vi "LidarROI.vi"(0 "x,y 배열":cluster{"x":dbl, "y":dbl}[](array[cluster])) -> (4 "ROI1":bool, 6 "ROI2":bool, 8 "ROI3":bool, 10 "왼쪽정적라이다스티어":dbl=144.0774265029782, 15 "오른쪽정적라이다스티어":dbl=-108.05806987723365)   [LabVIEW 2015]
panel:
  in  "x 场2":dbl=-100.0
  in  "y시작 3":dbl=500.0
  in  "y场 3":dbl=3000.0
  in  "x场 3":dbl=1400.0
  in  "x시작 3":dbl=100.0
  in  "x시작 2":dbl=-1400.0
  in  "y场 2":dbl=3000.0
  in  "y시작 2":dbl=500.0
  in  "x시작":dbl=-1400.0
  in  "x场":dbl=1400.0
  in  "y场":dbl=8000.0
  in  "y시작":dbl
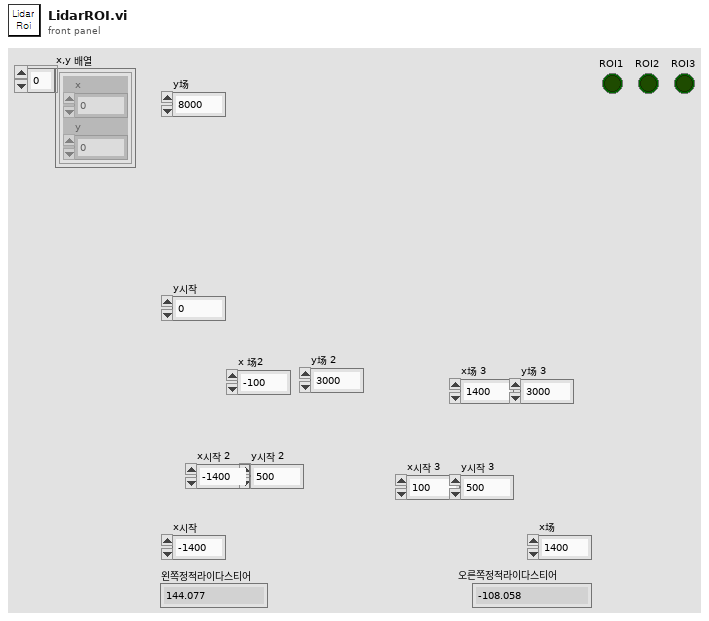
[diagram p1: front panel]
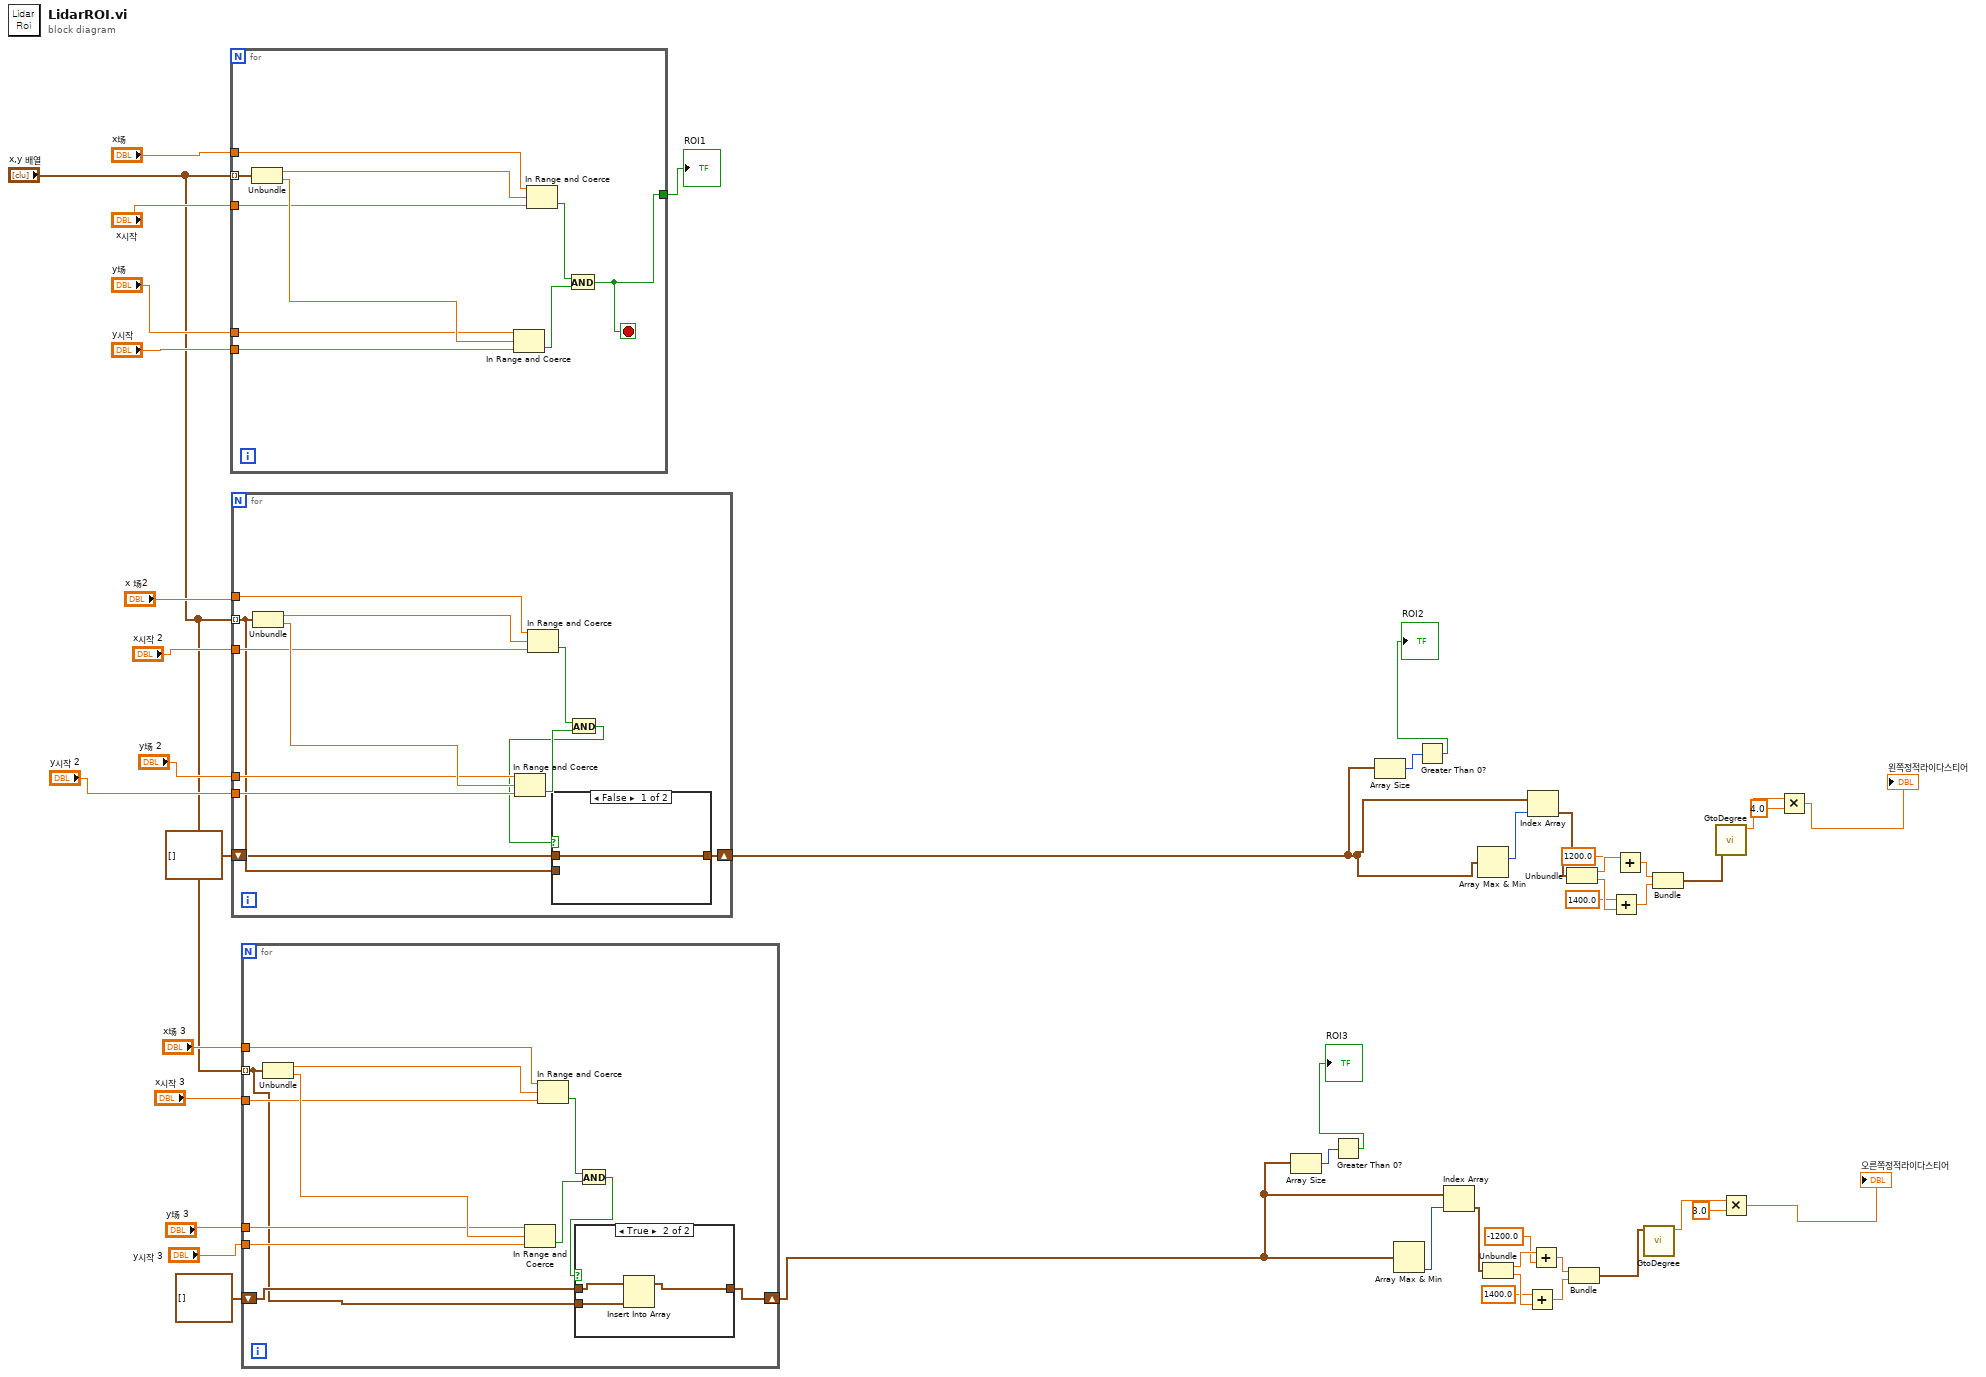
[diagram p0: block diagram]
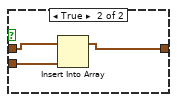
[diagram p3: hidden frame]
diagram:
  n1 = for {
    tunnel: "x,y 배열" -> [w56] mode=indexing
    tunnel: [w51] -> w46
    tunnel: "x场" -> [w50]
    tunnel: "x시작" -> [w49]
    tunnel: "y场" -> [w48]
    tunnel: "y시작" -> [w47]
    stop <- w51 stop-if-true
    n2 = Unbundle(w56) -> ("x"=w55:dbl, "y"=w52:dbl)
    n3 = In Range and Coerce(upper limit=w48, x=w52, lower limit=w47) -> (In Range?=w53:bool)  [unwired: 1 out]
    n4 = In Range and Coerce(upper limit=w50, x=w55, lower limit=w49) -> (In Range?=w54:bool)  [unwired: 1 out]
    n5 = And(x=w54, y=w53) -> (x .and. y?=w51:bool)
  }
  "ROI1" <- w46
  n6 = for {
    tunnel: "x,y 배열" -> [w59] mode=indexing
    tunnel: "x 场2" -> [w64]
    tunnel: "x시작 2" -> [w63]
    tunnel: "y场 2" -> [w62]
    tunnel: "y시작 2" -> [w61]
    shift-right: [w58] -> w31
    shift-left: cluster{"x":dbl, "y":dbl}[] [] -> [w57]
    n7 = Unbundle(w59) -> ("x"=w68:dbl, "y"=w65:dbl)
    n8 = In Range and Coerce(upper limit=w62, x=w65, lower limit=w61) -> (In Range?=w66:bool)  [unwired: 1 out]
    n9 = In Range and Coerce(upper limit=w64, x=w68, lower limit=w63) -> (In Range?=w67:bool)  [unwired: 1 out]
    n10 = And(x=w67, y=w66) -> (x .and. y?=w60:bool)
    n11 = case shown="False" w60 {
      tunnel: w59 -> [_ w72]
      tunnel: [w69 w71] -> w58
      tunnel: w57 -> [w69 w70]
      frame False {
      }
      frame True {
        n12 = Insert Into Array(array=w70, new element=w72) -> (w71:cluster{"x":dbl, "y":dbl}[])  [unwired: 1 in]
      }
    }
  }
  n13 = for {
    tunnel: "x,y 배열" -> [w73] mode=indexing
    tunnel: "x场 3" -> [w80]
    tunnel: "x시작 3" -> [w79]
    tunnel: "y场 3" -> [w78]
    tunnel: "y시작 3" -> [w77]
    shift-right: [w75] -> w12
    shift-left: cluster{"x":dbl, "y":dbl}[] [] -> [w74]
    n14 = Unbundle(w73) -> ("x"=w84:dbl, "y"=w81:dbl)
    n15 = In Range and Coerce(upper limit=w78, x=w81, lower limit=w77) -> (In Range?=w82:bool)  [unwired: 1 out]
    n16 = In Range and Coerce(upper limit=w80, x=w84, lower limit=w79) -> (In Range?=w83:bool)  [unwired: 1 out]
    n17 = And(x=w83, y=w82) -> (x .and. y?=w76:bool)
    n18 = case shown="True" w76 {
      tunnel: w73 -> [_ w88]
      tunnel: [w85 w87] -> w75
      tunnel: w74 -> [w85 w86]
      frame False {
      }
      frame True {
        n19 = Insert Into Array(array=w86, new element=w88) -> (w87:cluster{"x":dbl, "y":dbl}[])  [unwired: 1 in]
      }
    }
  }
  n20 = Array Size(array=w12) -> (size(s)=w15:i32)
  n21 = Greater Than 0?(x=w15) -> (x > 0?=→"ROI3":bool)
  n22 = Array Size(array=w31) -> (size(s)=w33:i32)
  n23 = Array Max & Min(array=w12) -> (min index (indices)=w9:i32)  [unwired: 3 out]
  n24 = Greater Than 0?(x=w33) -> (x > 0?=→"ROI2":bool)
  n25 = Index Array(array=w12, index=w9) -> (element=w16:cluster{"x":dbl, "y":dbl})
  n26 = Array Max & Min(array=w31) -> (max index (indices)=w30:i32)  [unwired: 3 out]
  n27 = Unbundle(w16) -> ("x"=w17:dbl, "y"=w20:dbl)
  n28 = Add(x=1400.0, y=w20) -> (x+y=w21:dbl)
  n29 = Index Array(array=w31, index=w30) -> (element=w29:cluster{"x":dbl, "y":dbl})
  n30 = Add(x=w17, y=-1200.0) -> (x+y=w18:dbl)
  n31 = Unbundle(w29) -> ("x"=w28:dbl, "y"=w24:dbl)
  n32 = Bundle(w18, w21) -> (w19:cluster{dbl, dbl})  [unwired: 1 in]
  n33 = Add(x=1400.0, y=w24) -> (x+y=w22:dbl)
  n34 = Add(x=w28, y=1200.0) -> (x+y=w26:dbl)
  n35 = call "GtoDegree.vi"("PathPointG"=w19) -> ("steer"=w5:dbl)  [unwired: 10 in]
  n36 = Bundle(w26, w22) -> (w1:cluster{dbl, dbl})  [unwired: 1 in]
  n37 = call "GtoDegree.vi"("PathPointG"=w1) -> ("steer"=w8:dbl)  [unwired: 10 in]
  n38 = Multiply(x=w5, y=3.0) -> (x*y=→"오른쪽정적라이다스티어":dbl)
  n39 = Multiply(x=w8, y=4.0) -> (x*y=→"왼쪽정적라이다스티어":dbl)
